vi "RGB_Invert.vi"(3 "Blue":i32[][](array[numeric]), 4 "Green":i32[][](array[numeric]), 5 "Red":i32[][](array[numeric])) -> (0 "Invert Blue":i32[][](array[numeric]), 1 "Invert Green":i32[][](array[numeric]), 2 "Invet Red":i32[][](array[numeric]))   [LabVIEW 2016]
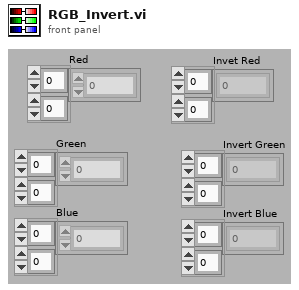
[diagram p1: front panel]
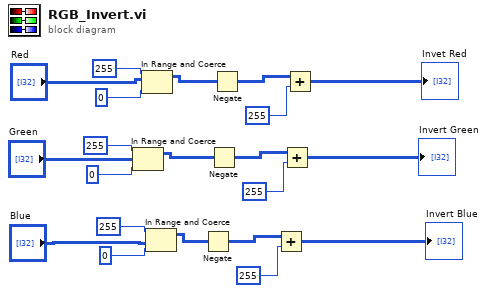
[diagram p0: block diagram]
diagram:
  n1 = In Range and Coerce(upper limit=255, x="Green", lower limit=0) -> (coerced(x)=w10:i32[][])  [unwired: 1 out]
  n2 = In Range and Coerce(upper limit=255, x="Red", lower limit=0) -> (coerced(x)=w11:i32[][])  [unwired: 1 out]
  n3 = In Range and Coerce(upper limit=255, x="Blue", lower limit=0) -> (coerced(x)=w7:i32[][])  [unwired: 1 out]
  n4 = Negate(x=w7) -> (-x=w17:i32[][])
  n5 = Negate(x=w10) -> (-x=w19:i32[][])
  n6 = Negate(x=w11) -> (-x=w21:i32[][])
  n7 = Add(x=w17, y=255) -> (x+y=→"Invert Blue":i32[][])
  n8 = Add(x=w19, y=255) -> (x+y=→"Invert Green":i32[][])
  n9 = Add(x=w21, y=255) -> (x+y=→"Invet Red":i32[][])
